vi "TWM Client Cmd Exec ADC Selfcalibration.vi"(7 "end of packet key":string="TWM:command:EndOfPacket", 8 "error in":errorcluster, 10 "timeout [s] (300)":dbl=300.0, 11 "handle":i32) -> (0 "error out":errorcluster, 3 "handle out":i32)   [LabVIEW 2020, in "TWM Client.lvlib"]
doc: "Executes digitizer selfcalibration routine, waits for completion. It is blocking operation, so the client and TWM will hangup untill operation is done or fails! Cannot be called while measurement is in progress!"
uses:
  TWM Client.lvlib
  octave/infolib/infolib.lvlib
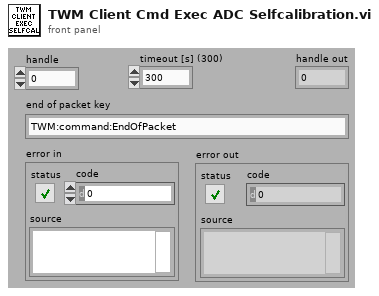
[diagram p1: front panel]
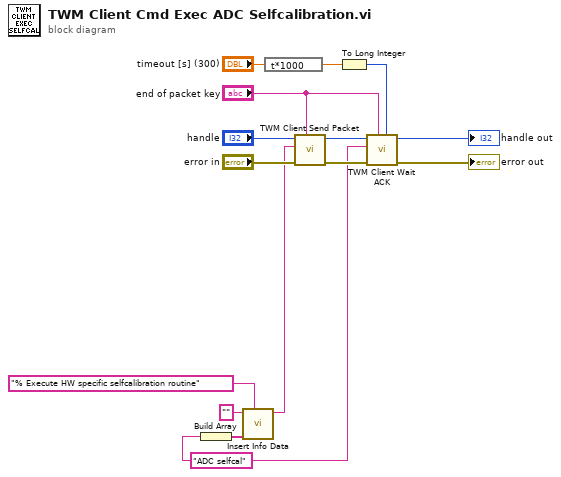
[diagram p0: block diagram]
diagram:
  w4 = "ADC selfcal" ("section name")
  n1 = Build Array(w4) -> (w12:string[])
  n2 = call "Insert Info Data.vi"("info data to insert"="% Execute HW specific selfcalibration routine", "sections"=w12, "info data"="") -> ("info data out"=w13:string)  [unwired: 7 in, 1 out]
  n3 = expression code="t*1000"("timeout [s] (300)") -> (w2:dbl)
  n4 = call "TWM Client Send Packet.vi"("end of packet key"="end of packet key", "error in"="error in", "command string"=w13, "handle"="handle") -> ("error out"=w10:errorcluster, "handle out"=w9:i32)  [unwired: 6 in]
  n5 = To Long Integer(number=w2) -> (32bit integer=w1:i32)
  n6 = call "TWM Client Wait ACK.vi"("timeout [ms] (3000)"=w1, "key string"="end of packet key", "error in"=w10, "command header"=w4, "handle"=w9) -> ("error out"=→"error out":errorcluster, "handle out"=→"handle out":i32)  [unwired: 5 in]
